vi "rqcBob Window Test - 2 SPD (Low Level Example).vi"() -> ()   [LabVIEW 2018]
uses:
  FPGA/rqcBob/Custom Controls/Pulse Train/rqcBob Pulse Train Config.ctl
  FPGA/rqcBob/Custom Controls/Pulse Train/rqcBob Pulse Train.Generation Mode.ctl
  FPGA/rqcBob/Custom Controls/Pulse Train/rqcBob Pulse Train.First Pulse Delay Mode.ctl
  FPGA/rqcBob/Custom Controls/rqcBob Modulator Config.ctl
  FPGA/rqcBob/Custom Controls/rqcBob Window Config.ctl
  Shared/Shared FPGA Lib/Shared Logic/Custom Controls/rqc Random Generator.parameters.ctl
  Shared/Shared FPGA Lib/Shared Logic/Custom Controls/rqc Random Generator.value type.ctl
  FPGA/rqcBob/Custom Controls/rqcBob Trigger Type.ctl
  <vilib>/FPGAPlugInAG/PCI-7811R/niLvFpga_Open_PCI-7811R.vi
  <vilib>/rvi/interface/common/dynamic/niFpgaDynamicAddResources.vi
  Low Level API/Configuration/Photon Detector/Detection FIFOs config/rqcBob Configure PD Detect FIFO (1PD PD1).vi
  Low Level API/Configuration/Photon Detector/Set PD window/rqcBob Configure SPD Detection Window (2PD).vi
  Low Level API/Read/Read PD Detection FIFO/rqcBob Read PD Detection FIFO (1PD PD1).vi
  <vilib>/FPGAPlugInAG/Dynamic/niLvFpga_Close_Dynamic.vi
  <vilib>/rvi/interface/nirviOpenFPGA/nirviOpenFPGA.xnode
  FPGA Bitfiles/rqcBob (FPGA) 7811 v 4.0.0.lvbitx
  <vilib>/rvi/interface/nirviCloseFPGA/nirviCloseFPGA.xnode
  <vilib>/Analysis/NI_AALBase.lvlib
panel:
  in  "Tab Control":enum32{"Main histograms", "Advanced histograms"}(tab)
  out "Num of Detections (1-st PD) vs Window":cluster{u32[], "appended array":dbl[]}(graph)={[0, 1, 2, 3, 4, 5, 6, 7, 8, 9, 10, 11, 12, 13, 14, 15, 16, 17, 18, 19, 20, 21, 22, 23, 24, 25, 26, 27, 28, 29, 30, 31, 32, 33, 34, 35, 36, 37, 38, 39], "appended array"=[0.0, 0.0, 0.0, 0.0, 0.0, 0.0, 0.0, 0.0, 0.0, 0.0, 0.0, 0.0, 0.0, 0.0, 0.0, 0.0, 0.0, 0.0, 0.0, 0.0, 0.0, 0.0, 0.0, 0.0, 0.0, 0.0, 0.0, 0.0, 0.0, 0.0, 0.0, 0.0, 0.0, 0.0, 0.0, 0.0, 0.0, 0.0, 0.0, 0.0]}
  out "Num of Detections (2-nd PD) vs Window":cluster{u32[], "appended array":dbl[]}(graph)={[0, 1, 2, 3, 4, 5, 6, 7, 8, 9, 10, 11, 12, 13, 14, 15, 16, 17, 18, 19, 20, 21, 22, 23, 24, 25, 26, 27, 28, 29, 30, 31, 32, 33, 34, 35, 36, 37, 38, 39], "appended array"=[0.0, 0.0, 0.0, 0.0, 0.0, 0.0, 0.0, 0.0, 0.0, 0.0, 0.0, 0.0, 0.0, 0.0, 0.0, 0.0, 0.0, 0.0, 0.0, 0.0, 0.0, 0.0, 0.0, 0.0, 0.0, 0.0, 0.0, 0.0, 0.0, 0.0, 0.0, 0.0, 0.0, 0.0, 0.0, 0.0, 0.0, 0.0, 0.0, 0.0]}
  out "Click Distribution By Period Number":T1(graph)
  out "PD1 Click Distribution":T1(graph)
  out "Modulation States Distribution":T1(graph)
  in  "modulator.clock delay":fxp<+,4,4> caption="PM Clock Delay (0-7) (in units of 40ns)"
  out "PD.detection window":u8=39 caption="SPD window scanned"
  in  "rndGen.parameters":T2={"value type"=enum."constant", "constant"=0, "num of levels"=4, "levels values"=[0, 0, 0, 0]} caption="Phase modulation value" {"num of levels" min=4 max=4 step=1}
  in  "window.config":T4 caption="Registration of detector clicks"
  in  "modulator.config":T5 caption="Phase modulation"
  in  "train.configuration":T6={"period"=0, "num of pulses"=0, "mode"=enum."train sequence.single", "num of trains"=0, "first pulse delay mode"=enum."every train", "first pulse delay"=55} caption="Pulsed laser configuration"
  in  "stop":bool
  out "Done":bool
  out "Progress":dbl(slide)=100.0 scale=0.0..100.0
  # "Bob configuration"
  # "Advanced parameters"
  # "Constant"
  # "Random"
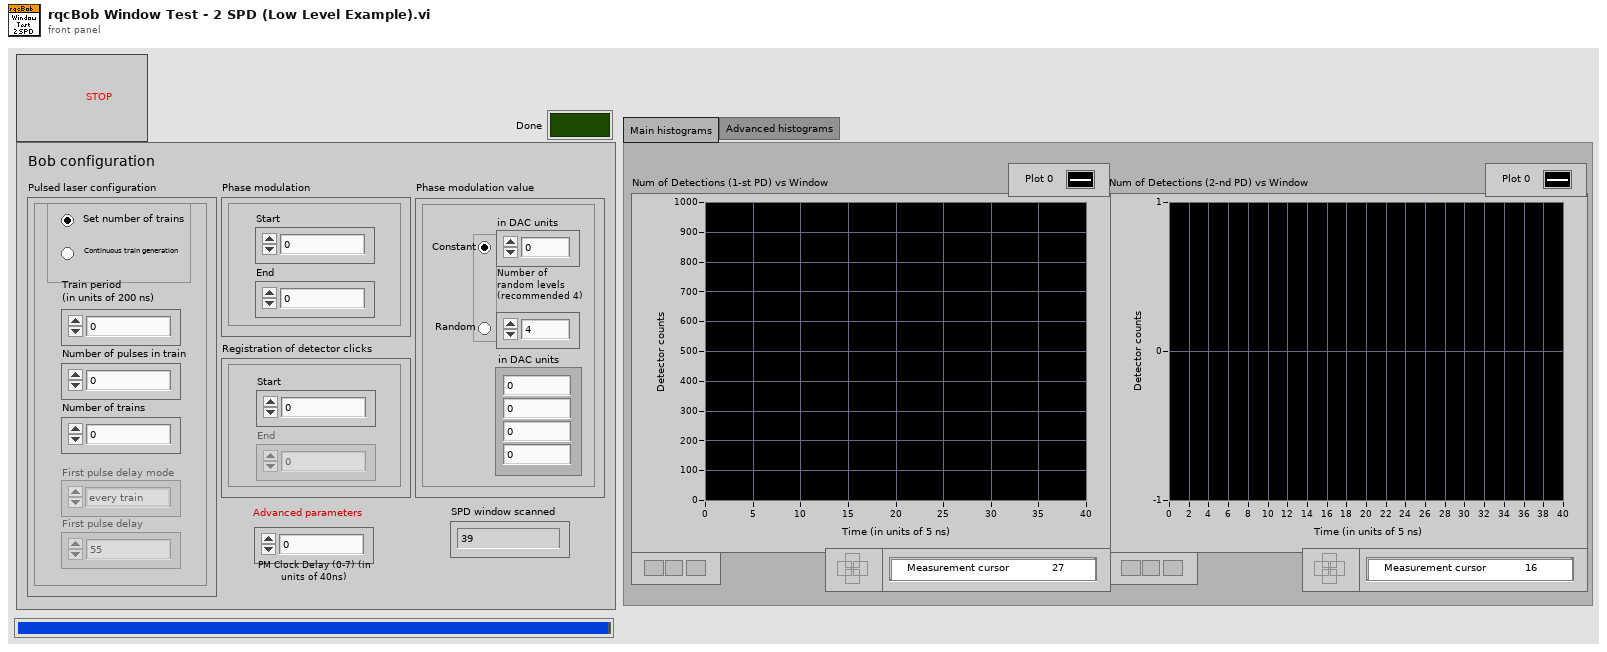
[diagram p1: front panel]
types:
  T1 = cluster{"X Values":dbl[], "Histogram: h(x)":i32[]}
  T2 = typedef "rqc Random Generator.parameters.ctl" = cluster{"value type":T3, "constant":u16, "num of levels":u16, "levels values":u16[]}
  T3 = typedef "rqc Random Generator.value type.ctl" = enum32{"random value", "constant"}
  T4 = typedef "rqcBob Window Config.ctl" = cluster{"window.open":u16, "window.close":u16}
  T5 = typedef "rqcBob Modulator Config.ctl" = cluster{"modulator.start":u16, "modulator.stop":u16}
  T6 = typedef "rqcBob Pulse Train Config.ctl" = cluster{"period":u16, "num of pulses":u16, "mode":T7, "num of trains":u16, "first pulse delay mode":T8, "first pulse delay":u16}
  T7 = typedef "rqcBob Pulse Train.Generation Mode.ctl" = enum32{"single train", "train sequence.single", "train sequence.wait for trigger", "continuous"}
  T8 = typedef "rqcBob Pulse Train.First Pulse Delay Mode.ctl" = enum8{"none", "every train", "first train"}
  T9 = typedef "rqcBob Trigger Type.ctl" = enum16{"software", "immediate", "DIO"}
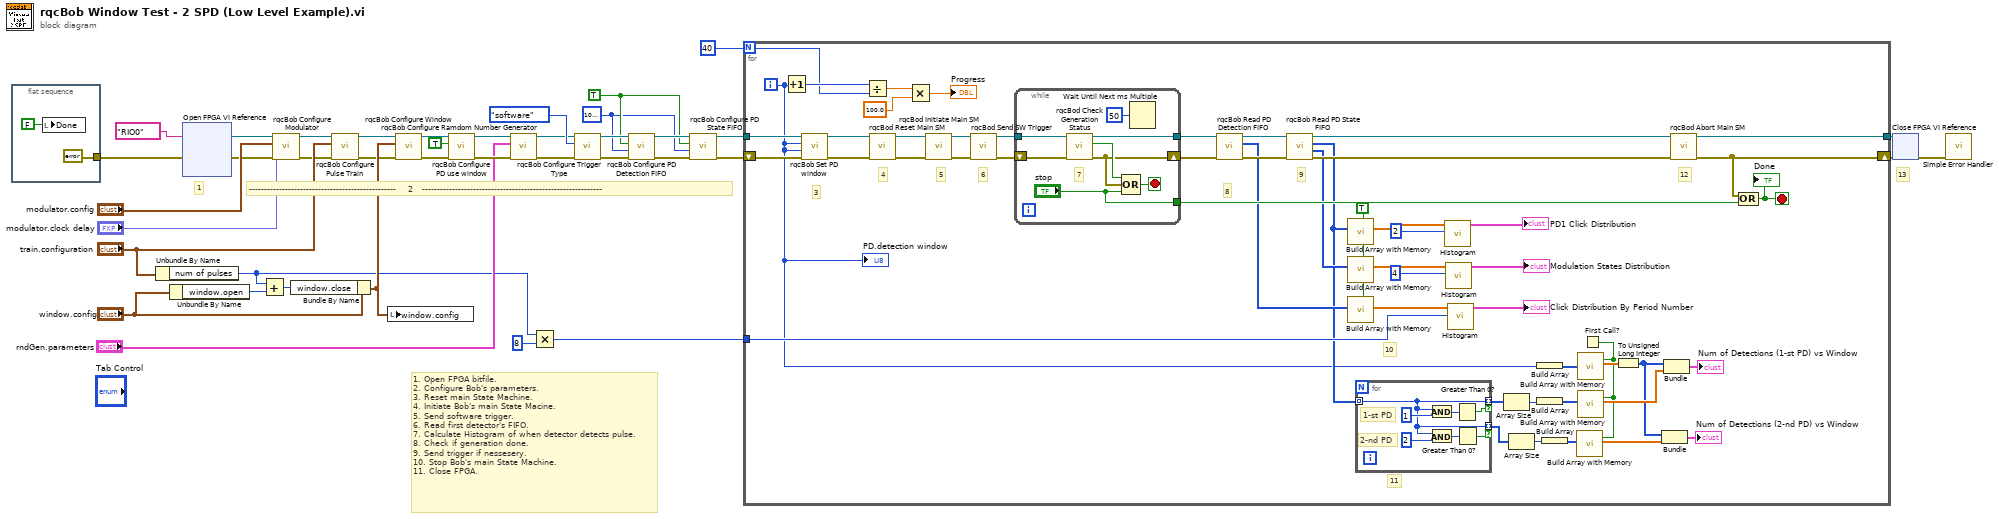
[diagram p0: block diagram]
diagram:
  w5 = TRUE ("SPD.detect fifo write enable")
  w4 = u32 1000000 ("SPD.detect fifo depth")
  # "13"
  # "1. Open FPGA bitfile.\n2. Configure Bob's parameters.\n3. Reset main State Machine.\n4. Initiate Bob's main State Macine.\n5. Send software trigger.\n6. Read first detector's FIFO.\n7. Calculate Histogram of when detector detects pulse.\n8. Check if generation done.\n9. Send trigger if nessesery.\n10. Stop Bob's main State Machine.\n11. Close FPGA."
  # "1"
  # "-------------------------------------------------    2   ------------------------------------------------------------"
  n1 = flat-sequence {
    tunnel: [errorcluster {"status"=FALSE, "code"=0, "source"=""} ("error in")] -> w36
    frame #0 {
      n2 = local write "Done"(FALSE ("Done")) -> ()
    }
  }
  n3 = Unbundle By Name("train.configuration") -> ("num of pulses"=w13:u16)
  n4 = Unbundle By Name("window.config") -> ("window.open"=w34:u16)
  n5 = xnode "Open FPGA VI Reference"("error in"=w36, "resource name"=tag "RIO0") -> ("FPGA VI Reference Out"=w10:refnum<k20>, "error out"=w9:errorcluster)
  n6 = Add(x=w13, y=w34) -> (x+y=w32:u16)
  n7 = call "rqcBob Configure Modulator.vi"("error in"=w9, "modulator.clock delay"="modulator.clock delay", "modulator.config"="modulator.config", "FPGA reference in"=w10) -> ("error out"=w25:errorcluster, "FPGA reference out"=w26:refnum<k20>)  [unwired: 6 in]
  n8 = Bundle By Name(cluster="window.config", "window.close"=w32) -> (w31:T4)
  n9 = call "rqcBob Configure Pulse Train.vi"("error in"=w25, "train.configuration"="train.configuration", "FPGA reference in"=w26) -> ("error out"=w27:errorcluster, "FPGA reference out"=w28:refnum<k20>)  [unwired: 6 in, 1 out]
  n10 = local write "window.config"(w31) -> ()
  n11 = call "rqcBob Configure Window.vi"("error in"=w27, "window.config"=w31, "FPGA reference in"=w28) -> ("error out"=w29:errorcluster, "FPGA reference out"=w30:refnum<k20>)  [unwired: 7 in]
  n12 = call "rqcBob Configure PD use window.vi"("error in"=w29, "PD.use window"=TRUE ("SPD.use detector window"), "FPGA reference in"=w30) -> ("error out"=w20:errorcluster, "FPGA reference out"=w21:refnum<k20>)  [unwired: 7 in]
  n13 = call "rqcBob Configure Ramdom Number Generator.vi"("error in"=w20, "rqcBob rndGen.parameters"="rndGen.parameters", "FPGA reference in"=w21) -> ("error out"=w18:errorcluster, "FPGA reference out"=w19:refnum<k20>)  [unwired: 7 in]
  n14 = Multiply(x=w13, y=u16 8) -> (x*y=w11:u16)
  n15 = call "rqcBob Configure Trigger Type.vi"("error in"=w18, "rqcBob Trigger Type"=rqcBob_Trigger_Type."software", "FPGA reference in"=w19) -> ("error out"=w3:errorcluster, "FPGA reference out"=w7:refnum<k20>)  [unwired: 7 in]
  n16 = call-poly "rqcBob Configure PD Detection FIFO.vi"("error in"=w3, "PD.detect fifo depth"=w4, "PD.detect fifo write enable"=w5, "FPGA reference in"=w7) -> ("error out"=w2:errorcluster, "FPGA reference out"=w6:refnum<k20>)  [unwired: 6 in]
  n17 = call "rqcBob Configure PD State FIFO.vi"("error in"=w2, "PD.state fifo depth"=w4, "PD.state fifo write enable"=w5, "FPGA reference in"=w6) -> ("error out"=w15:errorcluster, "FPGA reference out"=w16:refnum<k20>)  [unwired: 6 in]
  n18 = for {
    N: u8 40 ("SPD.detection cycle length") -> [w80]
    tunnel: w16 -> [w53]
    tunnel: [w88] -> w24
    shift-right: [w86] -> w23
    shift-left: w15 -> [w52]
    tunnel: w11 -> [w62]
    i -> [w49]
    stop <- w85 stop-if-true
    w58 = TRUE ("reset")
    # "4"
    # "11"
    # "10"
    # "9"
    # "8"
    # "12"
    # "6"
    # "5"
    # "3"
    n19 = Increment(x=w49) -> (x+1=w81:i32)
    n20 = call-poly "rqcBob Set PD window.vi"("error in"=w52, "PD2.detection window"=w49, "PD1.detection window"=w49, "FPGA reference in"=w53) -> ("error out"=w51:errorcluster, "FPGA reference out"=w50:refnum<k20>)  [unwired: 6 in]
    n21 = Divide(x=w81, y=w80) -> (x/y=w84:dbl)
    n22 = call "rqcBod Reset Main SM.vi"("error in"=w51, "FPGA reference in"=w50) -> ("error out"=w93:errorcluster, "FPGA reference out"=w94:refnum<k20>)  [unwired: 8 in]
    n23 = Multiply(x=w84, y=100.0) -> (x*y=→"Progress":dbl)
    n24 = call "rqcBod Initiate Main SM.vi"("error in"=w93, "FPGA reference in"=w94) -> ("error out"=w91:errorcluster, "FPGA reference out"=w92:refnum<k20>)  [unwired: 8 in]
    n25 = call "rqcBod Send SW Trigger.vi"("error in"=w91, "FPGA reference in"=w92) -> ("error out"=w89:errorcluster, "FPGA reference out"=w90:refnum<k20>)  [unwired: 8 in]
    n26 = while {
      tunnel: w90 -> [w103]
      shift-right: [w107] -> w78
      shift-left: w89 -> [w102]
      tunnel: [w108] -> w79
      tunnel: ["stop"] -> w87
      stop <- w106 stop-if-true
      # "7"
      n27 = call "rqcBod Check Generation Status.vi"("error in"=w102, "FPGA reference in"=w103) -> ("error out"=w107:errorcluster, "generation.done"=w109:bool, "FPGA reference out"=w108:refnum<k20>)  [unwired: 7 in]
      n28 = Compound Arithmetic op=OR(w109, w107, "stop") -> (w106:bool)
      n29 = Wait Until Next ms Multiple(millisecond multiple=u32 50) -> ()  [unwired: 1 out]
    }
    n30 = call-poly "rqcBob Read PD Detection FIFO.vi"("error in"=w78, "FPGA reference in"=w79) -> ("error out"=w76:errorcluster, "Data"=w64:u32[], "FPGA reference out"=w77:refnum<k20>)  [unwired: 6 in, 1 out]
    n31 = call "rqcBob Read PD State FIFO.vi"("error in"=w76, "FPGA reference in"=w77) -> ("error out"=w74:errorcluster, "PM Level"=w65:u8[], "SPD Number"=w61:u8[], "FPGA reference out"=w75:refnum<k20>)  [unwired: 6 in]
    n32 = call "Build Array with Memory.vi"("reset"=w58, "new array"=w61) -> ("appended array"=w67:dbl[])  [unwired: 9 in]
    n33 = call "Build Array with Memory.vi"("reset"=w58, "new array"=w65) -> ("appended array"=w66:dbl[])  [unwired: 9 in]
    n34 = call "Build Array with Memory.vi"("reset"=w58, "new array"=w64) -> ("appended array"=w63:dbl[])  [unwired: 9 in]
    n35 = for {
      tunnel: w61 -> [w96] mode=indexing
      tunnel: [w96] -> w60 mode=indexing if=w100
      tunnel: [w96] -> w46 mode=indexing if=w95
      # "2-nd PD"
      # "1-st PD"
      n36 = And(x=w96, y=u8 1) -> (x .and. y?=w99:u8)
      n37 = And(x=w96, y=u8 2) -> (x .and. y?=w97:u8)
      n38 = Greater Than 0?(x=w99) -> (x > 0?=w100:bool)
      n39 = Greater Than 0?(x=w97) -> (x > 0?=w95:bool)
    }
    n40 = call <vilib>:"Histogram.vi"("intervals"=2, "X"=w67) -> ("Histogram Graph"=→"PD1 Click Distribution":T1)  [unwired: 6 in, 3 out]
    n41 = call <vilib>:"Histogram.vi"("intervals"=4, "X"=w66) -> ("Histogram Graph"=→"Modulation States Distribution":T1)  [unwired: 6 in, 3 out]
    n42 = call <vilib>:"Histogram.vi"("intervals"=w62, "X"=w63) -> ("Histogram Graph"=→"Click Distribution By Period Number":T1)  [unwired: 6 in, 3 out]
    n43 = Array Size(array=w60) -> (size(s)=w59:i32)
    n44 = Array Size(array=w46) -> (size(s)=w47:i32)
    n45 = Build Array(w49) -> (w57:i32[])
    n46 = Build Array(w59) -> (w56:i32[])
    n47 = Build Array(w47) -> (w48:i32[])
    n48 = First Call?() -> (First Call?: T/F=w45:bool)
    n49 = call "Build Array with Memory.vi"("reset"=w45, "new array"=w48) -> ("appended array"=w42:dbl[])  [unwired: 9 in]
    n50 = call "Build Array with Memory.vi"("reset"=w45, "new array"=w57) -> ("appended array"=w55:dbl[])  [unwired: 9 in]
    n51 = call "Build Array with Memory.vi"("reset"=w45, "new array"=w56) -> ("appended array"=w54:dbl[])  [unwired: 9 in]
    n52 = To Unsigned Long Integer(number=w55) -> (unsigned 32bit integer=w43:u32[])
    n53 = Bundle(w43, "appended array"=w42) -> (→"Num of Detections (2-nd PD) vs Window":cluster{u32[], "appended array":dbl[]})  [unwired: 1 in]
    n54 = Bundle(w43, "appended array"=w54) -> (→"Num of Detections (1-st PD) vs Window":cluster{u32[], "appended array":dbl[]})  [unwired: 1 in]
    n55 = call "rqcBod Abort Main SM.vi"("error in"=w74, "FPGA reference in"=w75) -> ("error out"=w86:errorcluster, "FPGA reference out"=w88:refnum<k20>)  [unwired: 8 in]
    n56 = Compound Arithmetic op=OR(w86, w87) -> (w85:bool)
    "Done" <- w85
    "PD.detection window" <- w49
  }
  n57 = xnode "Close FPGA VI Reference"("FPGA VI Reference In"=w24, "error in"=w23) -> ("error out"=w22:errorcluster)
  n58 = call <vilib>:"Simple Error Handler.vi"("error in (no error)"=w22) -> ()  [unwired: 4 in, 5 out]
